vi "Sample & Graph Voltage From Chosen AI.vi"() -> ()   [LabVIEW 2018]
uses:
  <vilib>/DAQmx/read.llb/DAQmx Read (Analog DBL 1Chan 1Samp).vi
  <vilib>/DAQmx/create/channels.llb/DAQmx Create Channel (AI-Voltage-Basic).vi
  <vilib>/DAQmx/miscellaneous.llb/DAQmx Fill In Error Info.vi
panel:
  in  "Values to Display":dbl=100.0
  in  "physical channels":tag
  in  "stop":bool
  out "Waveform Chart":dbl(graph)
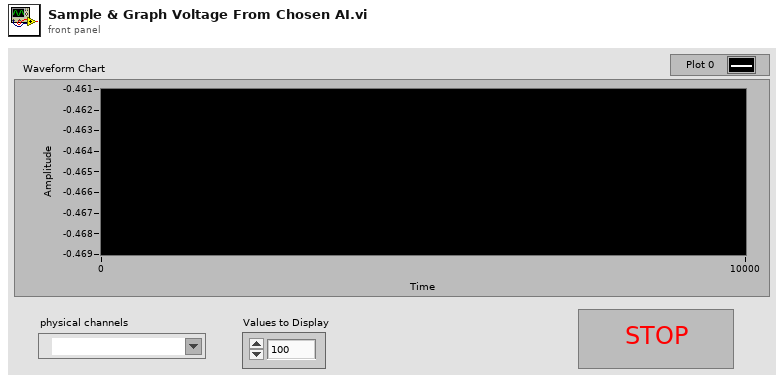
[diagram p1: front panel]
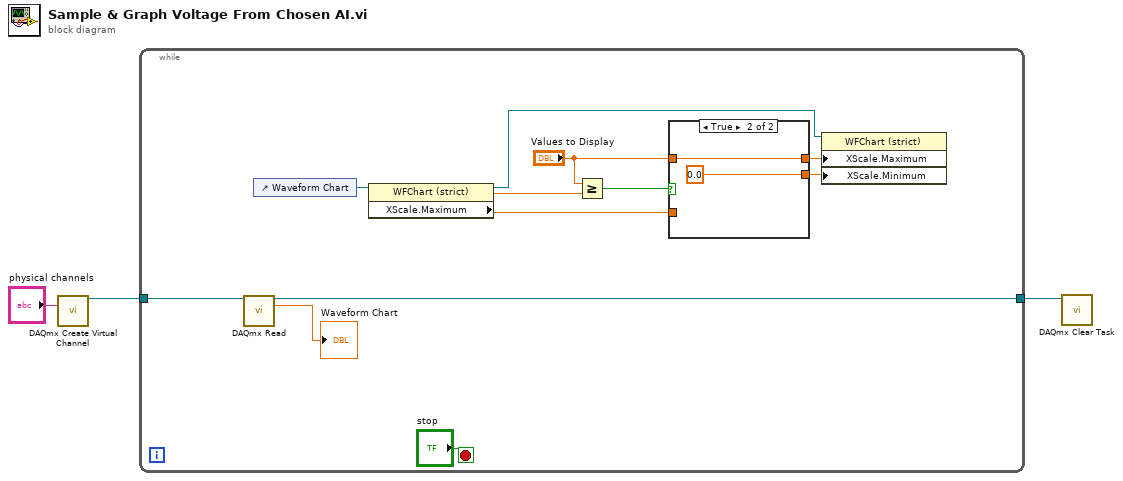
[diagram p0: block diagram]
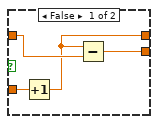
[diagram p2: hidden frame]
diagram:
  n1 = call-poly <vilib>:"DAQmx Create Virtual Channel.vi"("physical channels"="physical channels") -> ("task out"=w2:refnum<k21>)  [unwired: 13 in, 1 out]
  n2 = while {
    tunnel: w2 -> [w12]
    tunnel: [w11] -> w1
    stop <- "stop" stop-if-true
    n3 = call-poly <vilib>:"DAQmx Read.vi"("task/channels in"=w12) -> ("task out"=w11:refnum<k21>, "data"=→"Waveform Chart":dbl)  [unwired: 12 in, 1 out]
    n4 = control-ref of="Waveform Chart"() -> (w9:refnum<vi>)
    n5 = property on="Property Node" class="WFChart (strict)"(reference=w9) -> (reference out=w10:refnum<vi>, "XScale.Maximum"=w8:dbl)  [unwired: 1 in, 1 out]
    n6 = Greater Or Equal?(x="Values to Display", y=w8) -> (x >= y?=w7:bool)
    n7 = case shown="True" w7 {
      tunnel: "Values to Display" -> [w16 w20]
      tunnel: w8 -> [w18 _]
      tunnel: [w15 w20] -> w5
      tunnel: [w17 0.0] -> w4
      frame False {
        n8 = Increment(x=w18) -> (x+1=w15:dbl)
        n9 = Subtract(x=w15, y=w16) -> (x-y=w17:dbl)
      }
      frame True {
      }
    }
    n10 = property on="Property Node" class="WFChart (strict)"(reference=w10, "XScale.Maximum"=w5, "XScale.Minimum"=w4) -> ()  [unwired: 1 in, 2 out]
  }
  n11 = call <vilib>:"DAQmx Clear Task.vi"("task in"=w1) -> ()  [unwired: 14 in, 1 out]
